vi "Default Instrument Setup.vi"(8 "error in (no error)":errorcluster, 11 "VISA resource name":refnum<visa-resource-name>) -> (0 "error out":errorcluster, 3 "VISA resource name out":refnum<visa-resource-name>)   [LabVIEW 2015, in "Tektronix 7000 Series.lvlib"]
doc: "Sends a default command string to the instrument whenever a new VISA session is opened, or whenever the instrument is reset. Use this VI as a subVI for the Initialize and Reset VIs. Modifying this VI might cause these two VIs to operate incorrectly."
uses:
  Tektronix 7000 Series.lvlib
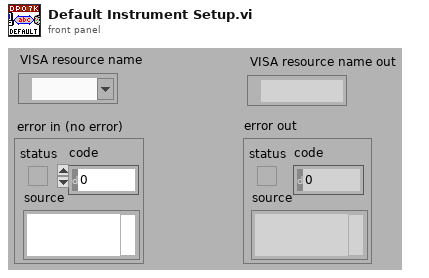
[diagram p1: front panel]
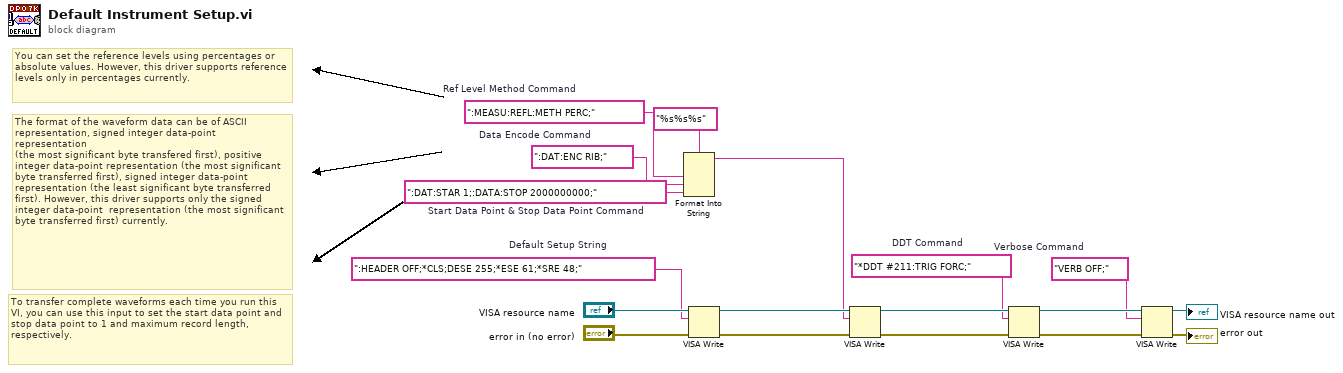
[diagram p0: block diagram]
diagram:
  w2 = ":DAT:STAR 1;:DATA:STOP 2000000000;"  # Start Data Point & Stop Data Point Command
  w1 = ":DAT:ENC RIB;"  # Data Encode Command
  w3 = ":HEADER OFF;*CLS;DESE 255;*ESE 61;*SRE 48;"  # Default Setup String
  w4 = "VERB OFF;"  # Verbose Command
  w9 = "*DDT #211:TRIG FORC;"  # DDT Command
  w16 = ":MEASU:REFL:METH PERC;"  # Ref Level Method Command
  # "To transfer complete waveforms each time you run this VI, you can use this input to set the start data point and stop data point to 1 and maximum record length, respectively."
  # "The format of the waveform data can be of ASCII\nrepresentation, signed integer data-point representation \n(the most significant byte transfered first), positive \ninteger data-point representation (the most significant \nbyte transferred first), signed integer data-point \nrepresentation (the least significant byte transferred first). However, this driver supports only the signed integer data-point  representation (the most significant byte transferred first) currently."
  # "You can set the reference levels using percentages or absolute values. However, this driver supports reference levels only in percentages currently."
  n1 = Format Into String(format string="%s%s%s", w16, w1, w2) -> (resulting string=w13:string)  [unwired: 2 in, 1 out]
  n2 = VISA Write(VISA resource name="VISA resource name", write buffer=w3, error in (no error)="error in (no error)") -> (VISA resource name out=w15:refnum<visa-resource-name>, error out=w14:errorcluster)  [unwired: 1 out]
  n3 = VISA Write(VISA resource name=w15, write buffer=w13, error in (no error)=w14) -> (VISA resource name out=w11:refnum<visa-resource-name>, error out=w10:errorcluster)  [unwired: 1 out]
  n4 = VISA Write(VISA resource name=w11, write buffer=w9, error in (no error)=w10) -> (VISA resource name out=w8:refnum<visa-resource-name>, error out=w7:errorcluster)  [unwired: 1 out]
  n5 = VISA Write(VISA resource name=w8, write buffer=w4, error in (no error)=w7) -> (VISA resource name out=→"VISA resource name out":refnum<visa-resource-name>, error out=→"error out":errorcluster)  [unwired: 1 out]
